vi "Pre Launch Init.vi"(11 "Chat Window in":refnum<class "Chat Window.lvclass">) -> (0 "error out":errorcluster, 3 "Chat Window out":refnum<class "Chat Window.lvclass">)   [LabVIEW 2020, in "Chat Window.lvlib" / "Chat Window.lvclass"]
doc: "(<B>Filename</B>: Actor Framework.lvlib:Actor.lvclass:Pre Launch Init.vi)\n\nDefines behavior that occurs after the Launch Nested Actor method is invoked but before the actor's Actor Core method begins running.\n\nBy default, this method does nothing. A descendant class may override it to define behavior."
uses:
  Chat Window.lvclass
  Chat Window.lvclass/Chat Window.ctl
  <vilib>/ActorFramework/Actor/Actor.lvclass
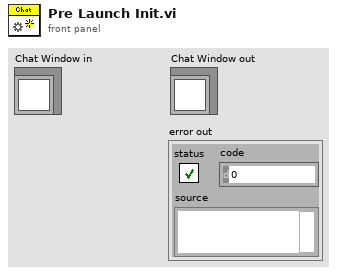
[diagram p1: front panel]
types:
  T1 = cluster{"Stop":refnum<user-event>, "Text":refnum<user-event>, "Connected":refnum<user-event>, "Number":refnum<user-event>, "echo":refnum<user-event>}
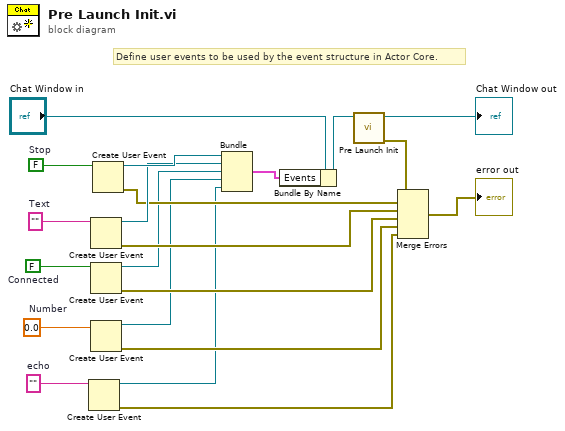
[diagram p0: block diagram]
diagram:
  w3 = ""  # echo
  w7 = 0.0  # Number
  w10 = FALSE  # Connected
  w18 = FALSE  # Stop
  w19 = ""  # Text
  # "Define user events to be used by the event structure in Actor Core."
  n1 = Create User Event(user event datatype=w3) -> (user event=w2:refnum<user-event>, error out=w1:errorcluster)  [unwired: 1 in]
  n2 = Create User Event(user event datatype=w19) -> (user event=w16:refnum<user-event>, error out=w13:errorcluster)  [unwired: 1 in]
  n3 = Create User Event(user event datatype=w10) -> (user event=w8:refnum<user-event>, error out=w9:errorcluster)  [unwired: 1 in]
  n4 = Create User Event(user event datatype=w7) -> (user event=w6:refnum<user-event>, error out=w4:errorcluster)  [unwired: 1 in]
  n5 = Create User Event(user event datatype=w18) -> (user event=w17:refnum<user-event>, error out=w14:errorcluster)  [unwired: 1 in]
  n6 = Bundle("Stop"=w17, "Text"=w16, "Connected"=w8, "Number"=w6, "echo"=w2) -> (w5:T1)  [unwired: 1 in]
  n7 = Bundle By Name(cluster="Chat Window in", "Events"=w5) -> (w15:refnum<class "Chat Window.lvclass">)
  n8 = call-parent "Pre Launch Init.vi"("Actor in"=w15) -> ("error out"=w12:errorcluster, "Actor out"=→"Chat Window out":refnum<class "Chat Window.lvclass">)  [unwired: 9 in]
  n9 = Merge Errors(w12, w14, w13, w9, w4, w1) -> (→"error out":errorcluster)
